vi "pco.labview_Live_CamRam_Example.vi"() -> ()   [LabVIEW 2020]
doc: "A short program to demonstrate the fundamentals of control and image acquision with the pco.camera series. The program records a sequence of images, with \"live\" updating, until the \"StopRecording\" button is pressed. Use ctrl-H for more help on the individual controls and indicators.\n\nCopyright 2004, 2010 The Cooke Corporation."
uses:
  CameraAccess.lvlib
  ImageSensor.lvlib
  TimingControl.lvlib
  Recorder.lvlib
  RecordingControl.lvlib
  CameraDescription.lvlib
  GeneralCameraControl.lvlib
panel:
  in  "wRamSegment":u16=1 caption="Ram Segment" min=1 max=4 step=1
  out "Recorded Images":u32
  in  "TriggerMode":u16(ring) items=["auto sequence"=0, "software trigger"=1, "external exposure start & software trigger"=2, "external exposure control"=3, "external synchronized"=4, "fast external exposure control"=5, "external CDS control"=6, "slow external exposure control"=7, "external synchronized HDSDI"=258]
  in  "Quit":bool
  out "Image":u16[][](graph)
  out "Error":errorcluster {"code" format="%x"}
  in  "Stop Record":bool
  out "Recording On":bool
  in  "roiY1":u16=2 max=0 step=1
  in  "roiX1":u16=2 max=0 step=1
  in  "roiY0":u16=1 min=1 step=1
  in  "roiX0":u16=1 min=1 step=1
  out "Image Height":u16
  out "Image Width":u16
  in  "Image Index":u32
  in  "dwImgCount":u32=10 caption="Required Number of Images" max=0
  in  "DelayTimeBase":u16(ring)=2 items=["nanoseconds", "microseconds", "milliseconds"]
  in  "ExposureTimeBase":u16(ring)=2 items=["nanoseconds", "microseconds", "milliseconds"]
  in  "Exposure":u32=10 min=1
  in  "Delay":u32
  in  "Rate":i32(ring) items=["Low", "High"]
  # "This example demonstrates the image acquisition with one camera with internal memory\nIt shows live display of the latest images during record. \nAfter record is stopped, the images can be addressed by index.\nNote that this example will not be fail save, i.e. doesnt react on errors, just handles them forward to the end\n\nUsage:\nSelect your required image count, ram segement and the camera setup before you start the program.\nOnce started, the camera will be opened and switched to ringbuffer mode.\nThe recorder will be created, initialized and images will be recorded and displayed automatically\nAfter the required number of images is recorded, acquisition is stopped. Or you can stop the record by pressing stop record at any time.\nAfter stopped, the image at the selected index will be read out\nTo finish the program click on Quit Application, this will force a free and delete of the recorder and a close camera\nYou can change your required ROI after and also during the record."
  # "pco.labview"
  # "Camera Setup"
  # "Recording Control"
  # "Parameters for image readout"
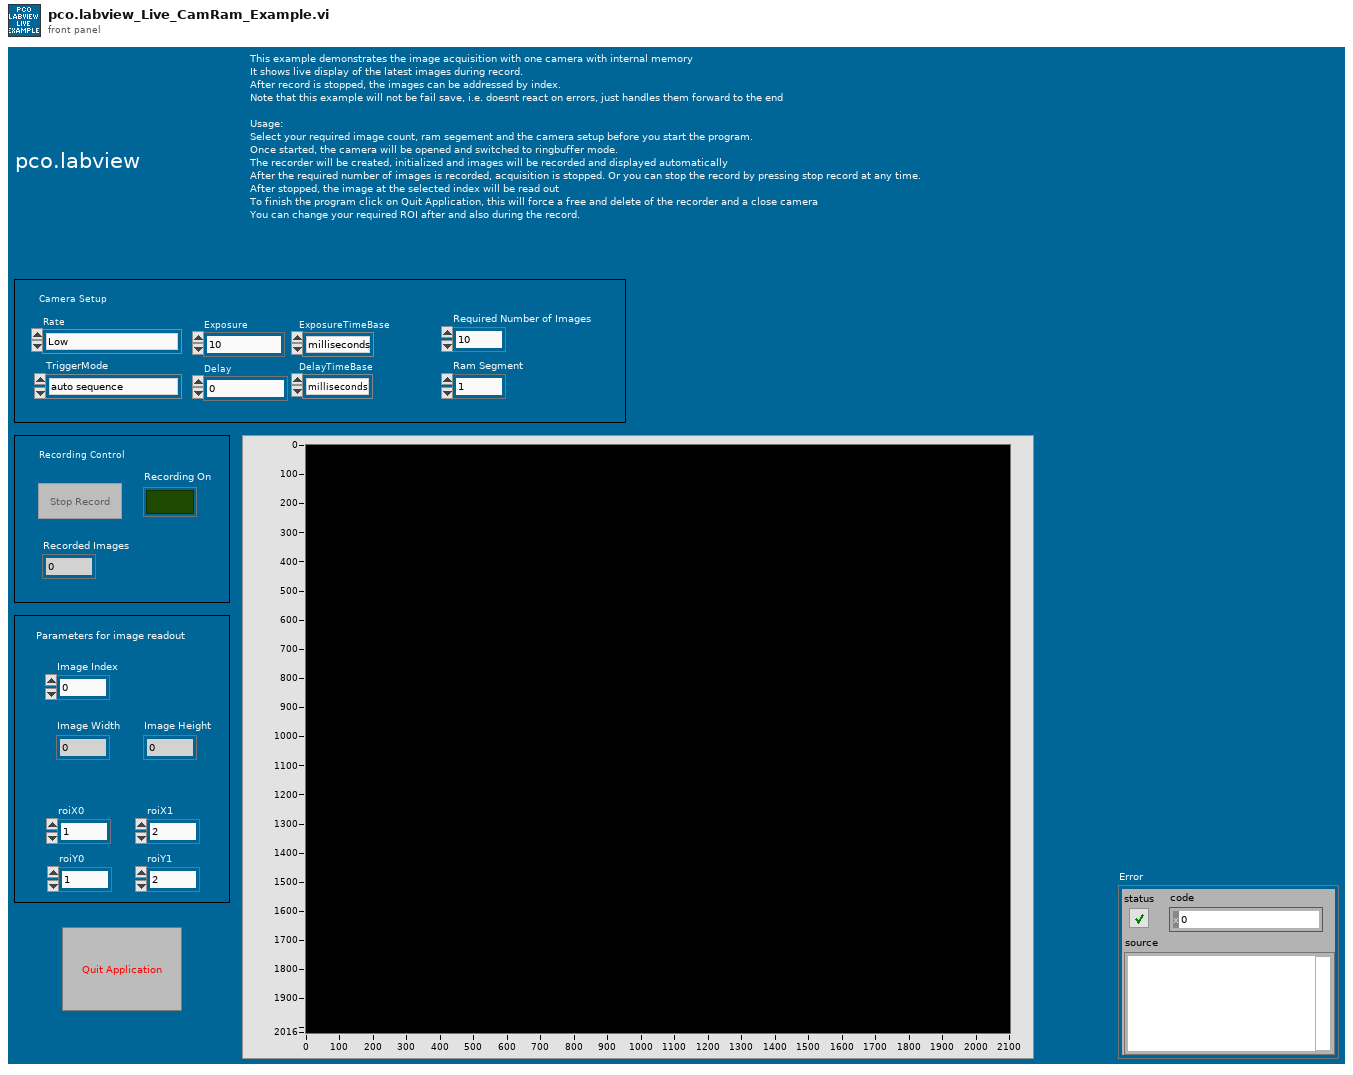
[diagram p1: front panel]
types:
  T1 = enum8{"Enabled", "Disabled", "Disabled and Grayed Out"}
  T2 = cluster{"wSensorTypeDESC":u16, "wSensorSubTypeDESC":u16, "wMaxHorzResStdDESC":u16, "wMaxVertResStdDESC":u16, "wMaxHorzResExtDESC":u16, "wMaxVertResExtDESC":u16, "wDynResDESC":u16, "wMaxBinHorzDESC":u16, "wBinHorzSteppingDESC":u16, "wMaxBinVertDESC":u16, "wBinVertSteppingDESC":u16, "wRoiHorStepsDESC":u16, "wRoiVertStepsDESC":u16, "wNumADCsDESC":u16, "wMinSizeHorzDESC":u16, "dwPixelRateDESC":u32[], "wConvFactDESC":u16[], "sCoolingSetpoints":i16[], "wSoftRoiHorStepsDESC":u16, "wSoftRoiVertStepsDESC":u16, "wIRDESC":u16, "wMinSizeVertDESC":u16, "dwMinDelayDESC":u32, "dwMaxDelayDESC":u32, "dwMinDelayStepDESC":u32, "dwMinExposureDESC":u32, "dwMaxExposureDESC":u32, "dwMinExposureStepDESC":u32, "dwMinDelayIRDESC":u32, "dwMaxDelayIRDESC":u32, "dwMinExposureIRDESC":u32, "dwMaxExposureIRDESC":u32, "wTimeTableDESC":u16, "wDoubleImageDESC":u16, "sMinCoolSetDESC":i16, "sMaxCoolSetDESC":i16, "sDefaultCoolSetDESC":i16, "wPowerDownModeDESC":u16, "wOffsetRegulationDESC":u16, "wColorPatternDESC":u16, "wPatternTypeDESC":u16, "wNumCoolingSetpoints":u16, "dwGeneralCapsDESC1":u32, "dwGeneralCapsDESC2":u32, "dwExtSyncFrequency":u32[], "dwGeneralCapsDESC3":u32, "dwGeneralCapsDESC4":u32}
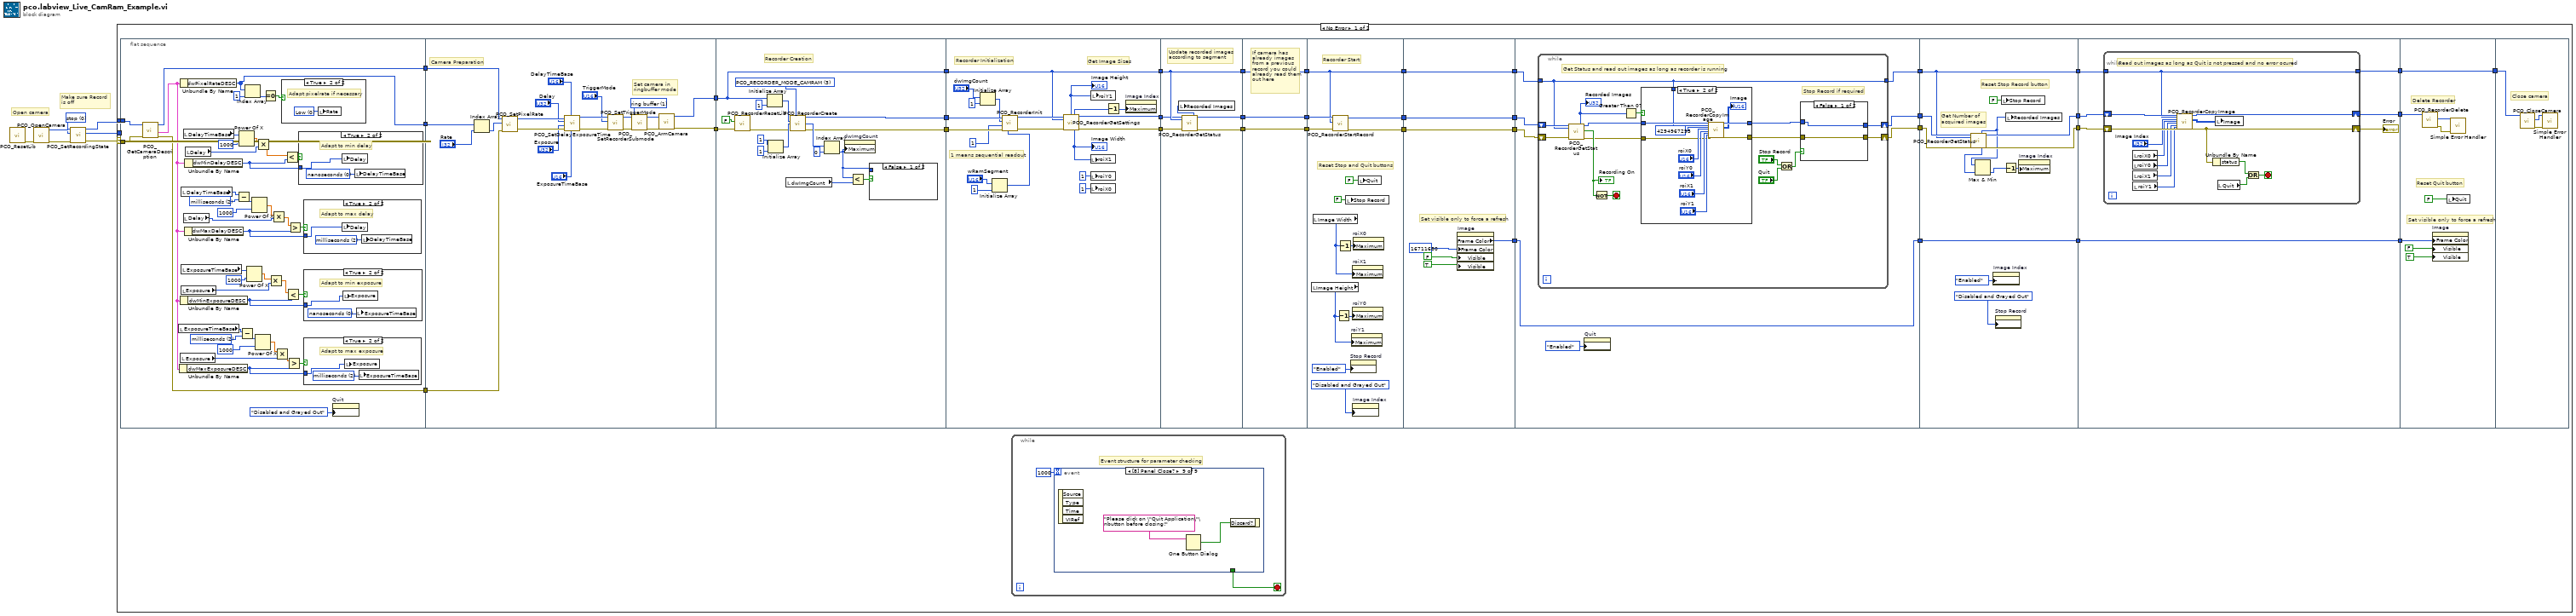
[diagram p0: block diagram]
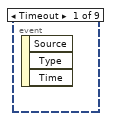
[diagram p2: hidden frame]
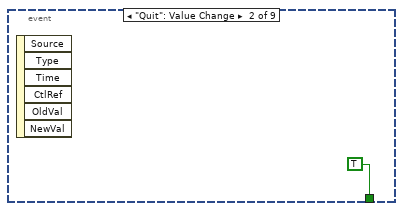
[diagram p3: hidden frame]
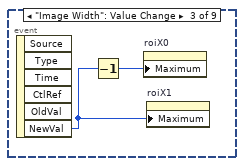
[diagram p4: hidden frame]
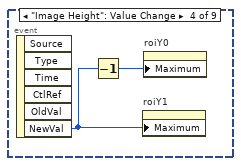
[diagram p5: hidden frame]
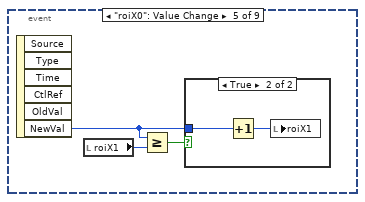
[diagram p6: hidden frame]
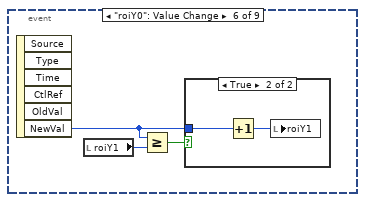
[diagram p8: hidden frame]
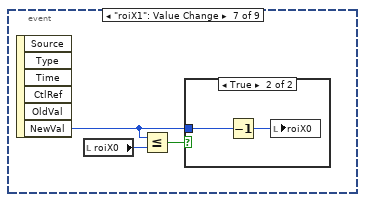
[diagram p10: hidden frame]
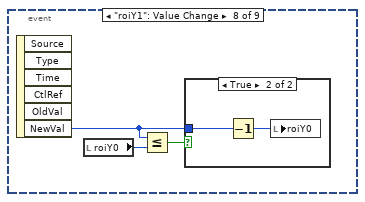
[diagram p12: hidden frame]
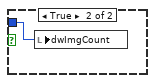
[diagram p19: hidden frame]
diagram:
  w4 = u16 0 items=["stop", "run"] ("wRecState")
  # "Make sure Record \nis off"
  # "Open camera"
  n1 = call "PCO_ResetLib.vi"() -> ("error out"=w7:errorcluster)  [unwired: 10 in, 1 out]
  n2 = call "PCO_OpenCamera.vi"("error in (no error)"=w7) -> ("error out"=w6:errorcluster, "ph out"=w5:u64)  [unwired: 8 in, 1 out]
  n3 = call "PCO_SetRecordingState.vi"("error in (no error)"=w6, "wRecState"=w4, "ph"=w5) -> ("error out"=w2:errorcluster, "ErrorMessage"=w1:i32, "ph out"=w3:u64)  [unwired: 6 in]
  n4 = case shown="No Error" w2 {
    selector: w2 -> [w44 w303]
    tunnel: w3 -> [w45 _]
    tunnel: w1 -> [_ w302]
    frame No Error {
      n5 = flat-sequence {
        tunnel: w44 -> [w113]
        tunnel: w45 -> [w114]
        tunnel: [w108] -> w19
        tunnel: [w116] -> w18
        tunnel: [w115] -> w17
        tunnel: [w126] -> w43
        tunnel: [w127] -> w42
        tunnel: w19 -> [w135]
        tunnel: w18 -> [w134]
        tunnel: w17 -> [w133]
        tunnel: w43 -> [w162]
        tunnel: w42 -> [w151]
        tunnel: [w153] -> w41
        tunnel: [w152] -> w40
        tunnel: [w151] -> w39
        tunnel: w41 -> [w184]
        tunnel: w40 -> [w183]
        tunnel: [w174] -> w16
        tunnel: [w175] -> w15
        tunnel: w39 -> [w173]
        tunnel: [w173] -> w14
        tunnel: w16 -> [w188]
        tunnel: [w186] -> w13
        tunnel: w15 -> [w187]
        tunnel: [w185] -> w11
        tunnel: w14 -> [w189]
        tunnel: [w189] -> w9
        tunnel: w13 -> [w193]
        tunnel: [w193] -> w12
        tunnel: w11 -> [w192]
        tunnel: [w192] -> w10
        tunnel: w9 -> [w191]
        tunnel: [w191] -> w8
        tunnel: w12 -> [w204]
        tunnel: w10 -> [w203]
        tunnel: [w202] -> w29
        tunnel: [w201] -> w27
        tunnel: w8 -> [w200]
        tunnel: [w200] -> w25
        tunnel: w29 -> [w207]
        tunnel: [w207] -> w28
        tunnel: w27 -> [w208]
        tunnel: [w208] -> w26
        tunnel: w25 -> [w209]
        tunnel: [w209] -> w24
        tunnel: [w210] -> w23
        tunnel: w28 -> [w221]
        tunnel: w26 -> [w219]
        tunnel: w24 -> [w220]
        tunnel: [w218] -> w37
        tunnel: [w217] -> w35
        tunnel: [w216] -> w33
        tunnel: w23 -> [w214]
        tunnel: [w214] -> w22
        tunnel: [w264] -> w38
        tunnel: w37 -> [w267]
        tunnel: [w265] -> w36
        tunnel: w35 -> [w266]
        tunnel: [w263] -> w34
        tunnel: w33 -> [w263]
        tunnel: w22 -> [w268]
        tunnel: [w268] -> w20
        tunnel: w38 -> [w276]
        tunnel: w36 -> [w275]
        tunnel: w34 -> [w274]
        tunnel: [w272] -> w32
        tunnel: [w271] -> w31
        tunnel: [w270] -> w21
        tunnel: w20 -> [w270]
        tunnel: w32 -> [w297]
        tunnel: w31 -> [w294]
        tunnel: [w294] -> w30
        tunnel: w21 -> [w291]
        tunnel: w30 -> [w301]
        frame #0 {
          w75 = u16 2 items=["nanoseconds", "microseconds", "milliseconds"] ("DelayTimeBase")
          w78 = u16 2 items=["nanoseconds", "microseconds", "milliseconds"] ("DelayTimeBase")
          n6 = call "PCO_GetCameraDescription.vi"("error in (no error)"=w113, "ph"=w114) -> ("error out"=w116:errorcluster, "strDescription"=w104:T2, "ph out"=w115:u64)  [unwired: 6 in, 1 out]
          n7 = local read "ExposureTimeBase"() -> (w76:u16)
          n8 = Unbundle By Name(w104) -> ("dwMaxExposureDESC"=w106:u32)
          n9 = Unbundle By Name(w104) -> ("dwPixelRateDESC"=w108:u32[])
          n10 = Unbundle By Name(w104) -> ("dwMinExposureDESC"=w105:u32)
          n11 = local read "Exposure"() -> (w83:u32)
          n12 = local read "Exposure"() -> (w81:u32)
          n13 = local read "DelayTimeBase"() -> (w77:u16)
          n14 = local read "ExposureTimeBase"() -> (w96:u16)
          n15 = local read "DelayTimeBase"() -> (w103:u16)
          n16 = local read "Delay"() -> (w88:u32)
          n17 = Unbundle By Name(w104) -> ("dwMaxDelayDESC"=w107:u32)
          n18 = Unbundle By Name(w104) -> ("dwMinDelayDESC"=w101:u32)
          n19 = local read "Delay"() -> (w99:u32)
          n20 = Subtract(x=w77, y=w78) -> (x-y=w92:i32)
          n21 = Power Of X(1:u32 1000 ("Delay"), 2:w103) -> (0:w100:dbl)
          n22 = Subtract(x=w76, y=w75) -> (x-y=w84:i32)
          n23 = Index Array(array=w108, index=1) -> (element=w110:u32)
          n24 = Power Of X(1:u32 1000 ("Delay"), 2:w96) -> (0:w95:dbl)
          n25 = Power Of X(1:u32 1000 ("Delay"), 2:w92) -> (0:w89:dbl)
          n26 = Power Of X(1:u32 1000 ("Delay"), 2:w84) -> (0:w86:dbl)
          n27 = Multiply(x=w100, y=w99) -> (x*y=w98:dbl)
          n28 = Equal To 0?(x=w110) -> (x = 0?=w109:bool)
          n29 = Multiply(x=w95, y=w81) -> (x*y=w80:dbl)
          n30 = Multiply(x=w89, y=w88) -> (x*y=w90:dbl)
          n31 = Multiply(x=w86, y=w83) -> (x*y=w82:dbl)
          n32 = case shown="True" w109 {
            frame False {
            }
            frame True {
              w125 = 0 items=["Low", "High"] ("Rate")
              # "Adapt pixelrate if necessary"
              n33 = local write "Rate"(w125) -> ()
            }
          }
          n34 = Less?(x=w98, y=w101) -> (x < y?=w97:bool)
          n35 = Less?(x=w80, y=w105) -> (x < y?=w79:bool)
          n36 = Greater?(x=w82, y=w106) -> (0:w87:bool)
          n37 = Greater?(x=w90, y=w107) -> (0:w93:bool)
          n38 = case shown="True" w97 {
            tunnel: w101 -> [_ w124]
            frame False {
            }
            frame True {
              w123 = u16 0 items=["nanoseconds", "microseconds", "milliseconds"] ("DelayTimeBase")
              # "Adapt to min delay"
              n39 = local write "Delay"(w124) -> ()
              n40 = local write "DelayTimeBase"(w123) -> ()
            }
          }
          n41 = case shown="True" w93 {
            tunnel: w107 -> [_ w122]
            frame False {
            }
            frame True {
              w121 = u16 2 items=["nanoseconds", "microseconds", "milliseconds"] ("DelayTimeBase")
              # "Adapt to max delay"
              n42 = local write "Delay"(w122) -> ()
              n43 = local write "DelayTimeBase"(w121) -> ()
            }
          }
          n44 = case shown="True" w79 {
            tunnel: w105 -> [_ w120]
            frame False {
            }
            frame True {
              w119 = u16 0 items=["nanoseconds", "microseconds", "milliseconds"] ("DelayTimeBase")
              # "Adapt to min exposure"
              n45 = local write "Exposure"(w120) -> ()
              n46 = local write "ExposureTimeBase"(w119) -> ()
            }
          }
          n47 = case shown="True" w87 {
            tunnel: w106 -> [_ w118]
            frame False {
            }
            frame True {
              w117 = u16 2 items=["nanoseconds", "microseconds", "milliseconds"] ("DelayTimeBase")
              # "Adapt to max exposure"
              n48 = local write "Exposure"(w118) -> ()
              n49 = local write "ExposureTimeBase"(w117) -> ()
            }
          }
          n50 = property on="Quit" class="Bool (strict)"("DisabledEnum"=T1."Disabled and Grayed Out" ("Disabled")) -> ()  [unwired: 2 in, 2 out]
        }
        frame #1 {
          w132 = u16 1 items=["sequence", "ring buffer"] ("wRecSubmode")
          # "Set camera in\nringbuffer mode"
          # "Camera Preparation"
          n51 = Index Array(array=w135, index="Rate") -> (element=w145:u32)
          n52 = call "PCO_SetPixelRate.vi"("error in (no error)"=w134, "dwPixelRate"=w145, "ph"=w133) -> ("error out"=w143:errorcluster, "ph out"=w144:u64)  [unwired: 6 in, 1 out]
          n53 = call "PCO_SetDelayExposureTime.vi"("wTimeBaseExposure"="ExposureTimeBase", "wTimeBaseDelay"="DelayTimeBase", "error in (no error)"=w143, "dwExposure"="Exposure", "dwDelay"="Delay", "ph"=w144) -> ("error out"=w137:errorcluster, "ph out"=w138:u64)  [unwired: 3 in, 1 out]
          n54 = call "PCO_SetTriggerMode.vi"("error in (no error)"=w137, "wTriggerMode"="TriggerMode", "ph"=w138) -> ("error out"=w128:errorcluster, "ph out"=w129:u64)  [unwired: 6 in, 1 out]
          n55 = call "PCO_SetRecorderSubmode.vi"("error in (no error)"=w128, "wRecSubmode"=w132, "ph"=w129) -> ("error out"=w131:errorcluster, "ph out"=w130:u64)  [unwired: 6 in, 1 out]
          n56 = call "PCO_ArmCamera.vi"("error in (no error)"=w131, "ph"=w130) -> ("error out"=w126:errorcluster, "ph out"=w127:u64)  [unwired: 7 in, 1 out]
        }
        frame #2 {
          w147 = u16 3 items=["PCO_RECORDER_MODE_FILE"=1, "PCO_RECORDER_MODE_MEMORY"=2, "PCO_RECORDER_MODE_CAMRAM"=3] ("dwRecMode")
          # "Recorder Creation"
          n57 = call "PCO_RecorderResetLib.vi"("error in (no error)"=w162, "bSilent"=FALSE) -> ("error out"=w154:errorcluster)  [unwired: 8 in, 1 out]
          n58 = Initialize Array(w151, 1 ("dimension size")) -> (w160:u64[])
          n59 = Initialize Array(u32 1 ("dimension size"), 1 ("dimension size")) -> (w157:u32[])
          n60 = local read "dwImgCount"() -> (w148:u32)
          n61 = call "PCO_RecorderCreate.vi"("wRecMode"=w147, "phCamArr"=w160, "dwImgDistributionArr"=w157, "error in (no error)"=w154) -> ("phRec out"=w152:u64, "dwMaxImgCountArr"=w156:u32[], "error out"=w153:errorcluster)  [unwired: 8 in, 1 out]
          n62 = Index Array(array=w156, index=0) -> (element=w149:u32)
          n63 = property on="dwImgCount" class="DigNum (strict)"("Maximum"=w149) -> ()  [unwired: 2 in, 2 out]
          n64 = Less?(x=w149, y=w148) -> (x < y?=w150:bool)
          n65 = case shown="False" w150 {
            tunnel: w149 -> [_ w164]
            frame False {
            }
            frame True {
              n66 = local write "dwImgCount"(w164) -> ()
            }
          }
        }
        frame #3 {
          # "1 means sequential readout"
          # "Get Image Sizes"
          # "Recorder Initialization"
          n67 = Initialize Array("dwImgCount", 1 ("dimension size")) -> (w180:u32[])
          n68 = Initialize Array("wRamSegment", 1 ("dimension size")) -> (w165:u16[])
          n69 = call "PCO_RecorderInit.vi"("wRamSegmentArr"=w165, "error in (no error)"=w184, "wType"=u16 1, "dwImgCountArr"=w180, "phRec"=w183) -> ("error out"=w179:errorcluster, "phRec out"=w178:u64)  [unwired: 4 in, 1 out]
          n70 = call "PCO_RecorderGetSettings.vi"("phRec"=w178, "phCam"=w173, "error in (no error)"=w179) -> ("wHeight"=w172:u16, "dwReqImgCount"=w169:u32, "phRec out"=w174:u64, "wWidth"=w171:u16, "error out"=w175:errorcluster)  [unwired: 4 in, 4 out]
          "Image Height" <- w172
          "Image Width" <- w171
          n71 = local write "roiX1"(w171) -> ()
          n72 = local write "roiY0"(u16 1 ("roiY0")) -> ()
          n73 = local write "roiX0"(u16 1 ("roiY0")) -> ()
          n74 = local write "roiY1"(w172) -> ()
          n75 = Decrement(x=w169) -> (x-1=w170:u32)
          n76 = property on="Image Index" class="DigNum (strict)"("Maximum"=w170) -> ()  [unwired: 2 in, 2 out]
        }
        frame #4 {
          # "Update recorded images\naccording to segment"
          n77 = call "PCO_RecorderGetStatus.vi"("phRec"=w188, "phCam"=w189, "error in (no error)"=w187) -> ("dwProcImgCount"=w190:u32, "phRec out"=w186:u64, "error out"=w185:errorcluster)  [unwired: 5 in, 9 out]
          n78 = local write "Recorded Images"(w190) -> ()
        }
        frame #5 {
          # "If camera has \nalready images\nfrom a previous\nrecord you could\nalready read them\nout here"
        }
        frame #6 {
          # "Reset Stop and Quit buttons"
          # "Recorder Start"
          n79 = local read "Image Height"() -> (w197:u16)
          n80 = local read "Image Width"() -> (w196:u16)
          n81 = call "PCO_RecorderStartRecord.vi"("error in (no error)"=w203, "phCam"=w200, "phRec"=w204) -> ("error out"=w202:errorcluster, "phRec out"=w201:u64)  [unwired: 6 in, 1 out]
          n82 = Decrement(x=w197) -> (x-1=w198:u16)
          n83 = Decrement(x=w196) -> (x-1=w199:u16)
          n84 = local write "Stop Record"(FALSE ("Stop Record")) -> ()
          n85 = property on="Stop Record" class="Bool (strict)"("DisabledEnum"=T1."Enabled" ("Disabled")) -> ()  [unwired: 2 in, 2 out]
          n86 = property on="roiY1" class="DigNum (strict)"("Maximum"=w197) -> ()  [unwired: 2 in, 2 out]
          n87 = property on="roiX1" class="DigNum (strict)"("Maximum"=w196) -> ()  [unwired: 2 in, 2 out]
          n88 = property on="roiY0" class="DigNum (strict)"("Maximum"=w198) -> ()  [unwired: 2 in, 2 out]
          n89 = property on="Image Index" class="DigNum (strict)"("DisabledEnum"=T1."Disabled and Grayed Out" ("Disabled")) -> ()  [unwired: 2 in, 2 out]
          n90 = property on="roiX0" class="DigNum (strict)"("Maximum"=w199) -> ()  [unwired: 2 in, 2 out]
          n91 = local write "Quit"(FALSE ("Stop")) -> ()
        }
        frame #7 {
          # "Set visible only to force a refresh"
          n92 = property on="Image" class="IntGraph (strict)"("Frame Color"=u32 16711680, "Visible"=FALSE, "Visible"=TRUE) -> ("Frame Color"=w210:u32)  [unwired: 2 in, 2 out]
        }
        frame #8 {
          n93 = while {
            tunnel: w220 -> [w226]
            shift-right: [w227] -> w217
            shift-left: w221 -> [w237]
            shift-right: [w228] -> w218
            shift-left: w219 -> [w233]
            tunnel: [w226] -> w216
            stop <- w232 stop-if-true
            # "Stop Record if required"
            # "Get Status and read out images as long as recorder is running"
            n94 = call "PCO_RecorderGetStatus.vi"("phRec"=w233, "phCam"=w226, "error in (no error)"=w237) -> ("dwProcImgCount"=w222:u32, "phRec out"=w235:u64, "bIsRunning"=w236:bool, "error out"=w234:errorcluster)  [unwired: 5 in, 8 out]
            "Recording On" <- w236
            "Recorded Images" <- w222
            n95 = Not(x=w236) -> (.not. x?=w232:bool)
            n96 = Greater Than 0?(x=w222) -> (x > 0?=w223:bool)
            n97 = case shown="True" w223 {
              tunnel: w235 -> [w239 w250]
              tunnel: w234 -> [w238 w244]
              tunnel: [w239 w243] -> w231
              tunnel: [w238 w242] -> w230
              tunnel: w226 -> [_ w241]
              frame False {
              }
              frame True {
                n98 = call "PCO_RecorderCopyImage.vi"("phRec"=w250, "phCam"=w241, "dwImgIdx"=u32 4294967295, "wRoiX0"="roiX0", "wRoiY0"="roiY0", "wRoiX1"="roiX1", "wRoiY1"="roiY1", "error in (no error)"=w244) -> ("phRec out"=w243:u64, "wImgBuf"=→"Image":u16[][], "error out"=w242:errorcluster)  [unwired: 13 in, 4 out]
              }
            }
            n99 = Or(x="Stop Record", y="Quit") -> (x .or. y?=w229:bool)
            n100 = case shown="False" w229 {
              tunnel: w231 -> [w252 w256]
              tunnel: w230 -> [w251 w255]
              tunnel: [w252 w253] -> w228
              tunnel: [w251 w254] -> w227
              frame False {
              }
              frame True {
                n101 = call "PCO_RecorderStopRecord.vi"("error in (no error)"=w255, "phRec"=w256) -> ("error out"=w254:errorcluster, "phRec out"=w253:u64)  [unwired: 7 in, 1 out]
              }
            }
          }
          n102 = property on="Quit" class="Bool (strict)"("DisabledEnum"=T1."Enabled" ("Disabled")) -> ()  [unwired: 2 in, 2 out]
        }
        frame #9 {
          # "Get Number of \nacquired images"
          # "Reset Stop Record button"
          n103 = call "PCO_RecorderGetStatus.vi"("phRec"=w267, "phCam"=w263, "error in (no error)"=w266) -> ("dwProcImgCount"=w260:u32, "dwReqImgCount"=w259:u32, "phRec out"=w264:u64, "error out"=w265:errorcluster)  [unwired: 5 in, 8 out]
          n104 = Max & Min(x=w260, y=w259) -> (min(x,y)=w261:u32)  [unwired: 1 out]
          n105 = property on="Image Index" class="DigNum (strict)"("DisabledEnum"=T1."Enabled" ("Disabled")) -> ()  [unwired: 2 in, 2 out]
          n106 = property on="Stop Record" class="Bool (strict)"("DisabledEnum"=T1."Disabled and Grayed Out" ("Disabled")) -> ()  [unwired: 2 in, 2 out]
          n107 = local write "Stop Record"(FALSE ("Stop Record")) -> ()
          n108 = Decrement(x=w261) -> (x-1=w262:u32)
          n109 = local write "Recorded Images"(w260) -> ()
          n110 = property on="Image Index" class="DigNum (strict)"("Maximum"=w262) -> ()  [unwired: 2 in, 2 out]
        }
        frame #10 {
          n111 = while {
            shift-right: [w278] -> w273
            shift-left: w275 -> [w287]
            shift-right: [w279] -> w272
            shift-left: w276 -> [w286]
            tunnel: w274 -> [w277]
            tunnel: [w277] -> w271
            stop <- w288 stop-if-true
            # "Read out images as long as Quit is not pressed and no error ocured"
            n112 = local read "roiX0"() -> (w284:u16)
            n113 = local read "roiY0"() -> (w283:u16)
            n114 = local read "roiX1"() -> (w282:u16)
            n115 = local read "roiY1"() -> (w281:u16)
            n116 = call "PCO_RecorderCopyImage.vi"("phRec"=w286, "phCam"=w277, "dwImgIdx"="Image Index", "wRoiX0"=w284, "wRoiY0"=w283, "wRoiX1"=w282, "wRoiY1"=w281, "error in (no error)"=w287) -> ("phRec out"=w279:u64, "wImgBuf"=w280:u16[][], "error out"=w278:errorcluster)  [unwired: 13 in, 4 out]
            n117 = Unbundle By Name(w278) -> ("status"=w290:bool)
            n118 = local write "Image"(w280) -> ()
            n119 = local read "Quit"() -> (w289:bool)
            n120 = Or(x=w290, y=w289) -> (x .or. y?=w288:bool)
          }
          "Error" <- w273
        }
        frame #11 {
          # "Set visible only to force a refresh"
          # "Delete Recorder"
          # "Reset Quit button"
          n121 = call "PCO_RecorderDelete.vi"("phRec"=w297) -> ("error out"=w295:errorcluster, "ErrorMessage"=w296:i32)  [unwired: 9 in]
          n122 = property on="Image" class="IntGraph (strict)"("Frame Color"=w291, "Visible"=FALSE, "Visible"=TRUE) -> ()  [unwired: 2 in, 2 out]
          n123 = local write "Quit"(FALSE ("Stop Record")) -> ()
          n124 = call "Simple Error Handler.vi"("error code (no error:0)"=w296, "error in (no error)"=w295) -> ()  [unwired: 3 in, 5 out]
        }
        frame #12 {
          # "Close camera"
          n125 = call "PCO_CloseCamera.vi"("ph"=w301) -> ("error out"=w299:errorcluster, "ErrorMessage"=w300:i32)  [unwired: 9 in]
          n126 = call "Simple Error Handler.vi"("error code (no error:0)"=w300, "error in (no error)"=w299) -> ()  [unwired: 3 in, 5 out]
        }
      }
      n127 = while {
        stop <- w46 stop-if-true
        # "Event structure for parameter checking"
        n128 = event shown="[8] Panel Close?" {
          selector: _ -> [_ _ _ _ _ _ _ _ _]
          dyn-events: _ -> [_ _ _ _ _ _ _ _ _]
          timeout: 1000 -> [_ _ _ _ _ _ _ _ _]
          tunnel: [_ TRUE _ _ _ _ _ _ _] -> w46
          event Timeout {
            n129 = event-data() -> ()  [unwired: 1 in, 3 out]
          }
          event "Quit": Value Change {
            n130 = event-data() -> ()  [unwired: 1 in, 6 out]
          }
          event "Image Width": Value Change {
            n131 = event-data() -> ("NewVal"=w49:u16)  [unwired: 1 in, 5 out]
            n132 = Decrement(x=w49) -> (x-1=w50:u16)
            n133 = property on="roiX0" class="DigNum (strict)"("Maximum"=w50) -> ()  [unwired: 2 in, 2 out]
            n134 = property on="roiX1" class="DigNum (strict)"("Maximum"=w49) -> ()  [unwired: 2 in, 2 out]
          }
          event "Image Height": Value Change {
            n135 = event-data() -> ("NewVal"=w51:u16)  [unwired: 1 in, 5 out]
            n136 = Decrement(x=w51) -> (x-1=w52:u16)
            n137 = property on="roiY1" class="DigNum (strict)"("Maximum"=w51) -> ()  [unwired: 2 in, 2 out]
            n138 = property on="roiY0" class="DigNum (strict)"("Maximum"=w52) -> ()  [unwired: 2 in, 2 out]
          }
          event "roiX0": Value Change {
            n139 = event-data() -> ("NewVal"=w53:u16)  [unwired: 1 in, 5 out]
            n140 = local read "roiX1"() -> (w55:u16)
            n141 = Greater Or Equal?(x=w53, y=w55) -> (x >= y?=w54:bool)
            n142 = case shown="True" w54 {
              tunnel: w53 -> [_ w57]
              frame False {
              }
              frame True {
                n143 = Increment(x=w57) -> (x+1=w56:u16)
                n144 = local write "roiX1"(w56) -> ()
              }
            }
          }
          event "roiY0": Value Change {
            n145 = event-data() -> ("NewVal"=w58:u16)  [unwired: 1 in, 5 out]
            n146 = local read "roiY1"() -> (w60:u16)
            n147 = Greater Or Equal?(x=w58, y=w60) -> (x >= y?=w59:bool)
            n148 = case shown="True" w59 {
              tunnel: w58 -> [_ w62]
              frame False {
              }
              frame True {
                n149 = Increment(x=w62) -> (x+1=w61:u16)
                n150 = local write "roiY1"(w61) -> ()
              }
            }
          }
          event "roiX1": Value Change {
            n151 = event-data() -> ("NewVal"=w63:u16)  [unwired: 1 in, 5 out]
            n152 = local read "roiX0"() -> (w65:u16)
            n153 = Less Or Equal?(x=w63, y=w65) -> (x <= y?=w64:bool)
            n154 = case shown="True" w64 {
              tunnel: w63 -> [_ w67]
              frame False {
              }
              frame True {
                n155 = Decrement(x=w67) -> (x-1=w66:u16)
                n156 = local write "roiX0"(w66) -> ()
              }
            }
          }
          event "roiY1": Value Change {
            n157 = event-data() -> ("NewVal"=w68:u16)  [unwired: 1 in, 5 out]
            n158 = local read "roiY0"() -> (w70:u16)
            n159 = Less Or Equal?(x=w68, y=w70) -> (x <= y?=w69:bool)
            n160 = case shown="True" w69 {
              tunnel: w68 -> [_ w72]
              frame False {
              }
              frame True {
                n161 = Decrement(x=w72) -> (x-1=w71:u16)
                n162 = local write "roiY0"(w71) -> ()
              }
            }
          }
          event Panel Close? {
            n163 = event-data() -> ()  [unwired: 1 in, 4 out]
            n164 = One Button Dialog(message="Please click on \"Quit Application\"\nbutton before closing!") -> (true=w73:bool)  [unwired: 1 in]
            n165 = event-data("Discard?"=w73) -> ()  [unwired: 1 in, 1 out]
          }
        }
      }
    }
    frame Error {
      n166 = call "Simple Error Handler.vi"("error code (no error:0)"=w302, "error in (no error)"=w303) -> ()  [unwired: 3 in, 5 out]
    }
  }
